vi "User Drivetrain Control.vi"(8 "reinitialize":bool) -> ()   [LabVIEW 2011]
uses:
  <vilib>/Rock Robotics/WPI/RobotDrive/WPI_RobotDriveArcadeDrive_Standard(NoSaturation).vi
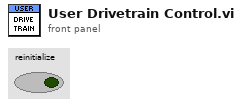
[diagram p1: front panel]
types:
  T1 = typedef "WPI_JoystickDevRef.ctl" = cluster{"Device":T2}
  T2 = typedef "WPI_JoystickDeviceEnum.ctl" = enum16{"USB 1", "USB 2", "USB 3", "USB 4", "Kinect 1", "Kinect 2"}
  T3 = typedef "WPI_JoystickButtonState.ctl" = cluster{"Button 1":bool, "Button 2":bool, "Button 3":bool, "Button 4":bool, "Button 5":bool, "Button 6":bool, "Button 7":bool, "Button 8":bool, "Button 9":bool, "Button 10":bool, "Button 11":bool, "Button 12":bool}
  T4 = cluster{"axis 1 (x)":dbl, "axis 2 (y)":dbl, "axis 3 (throttle)":dbl, "axis 4":dbl, "axis 5":dbl, "axis 6":dbl}
  T5 = typedef "WPI_RobotDriveDevRef.ctl" = cluster{"DevStatus":errorcluster, "Motors[]":T6[], "Square Inputs":bool, "Max Output":dbl, "Isochronous":bool}
  T6 = typedef "WPI_MotorControlDeviceRef.ctl" = cluster{"DeviceStatus":errorcluster, "Type":enum16{"PWM", "CAN"}, "PWM":cluster{"Digital Module":T7, "PWM Channel":T8, "DeadBand":T9}, "CAN":cluster{"Device Number":u8, "Control Mode":T10, "Semaphore":T11, "Max Vout":dbl}, "Invert":bool, "TransformRef":T12, "InvTransformRef":T12}
  T7 = typedef "FPGA_TypedefDigitalModule.ctl" = enum16{"Digital Module 1", "Digital Module 2"}
  T8 = typedef "FPGA_DIOPWMChannel.ctl" = enum8{"PWM 1", "PWM 2", "PWM 3", "PWM 4", "PWM 5", "PWM 6", "PWM 7", "PWM 8", "PWM 9", "PWM 10", "Invalid"}
  T9 = typedef "WPI_PWMDeadband.ctl" = cluster{"Name":string, "maxPositivePwm":i32, "minPositivePwm":i32, "centerPwm":i32, "maxNegativePwm":i32, "minNegativePwm":i32, "angularRange":u16}
  T10 = typedef "WPI_CANJaguar_ControlMode.ctl" = enum8{"Percent VBus", "Current", "Speed", "Position", "Voltage"}
  T11 = typedef "Semaphore RefNum" = refnum<k1>
  T12 = typedef "WPI_PWMTransform_ConPane.ctl" = refnum<vi>
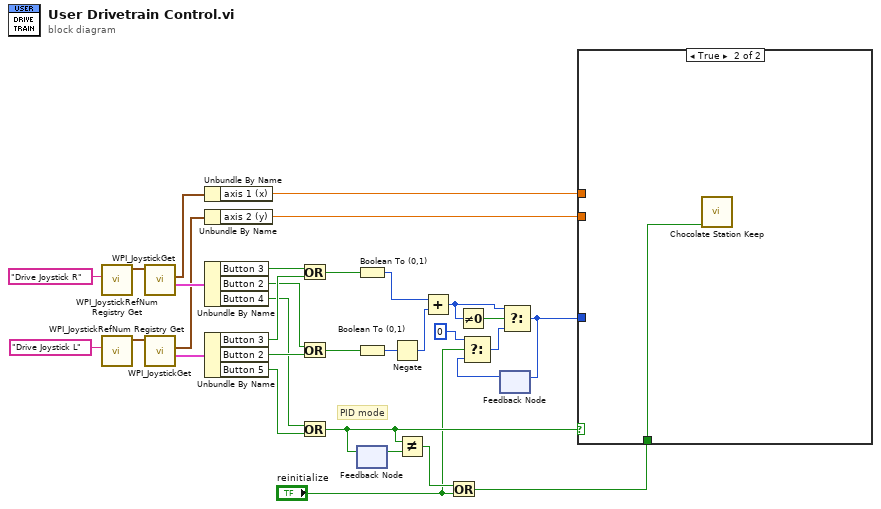
[diagram p0: block diagram]
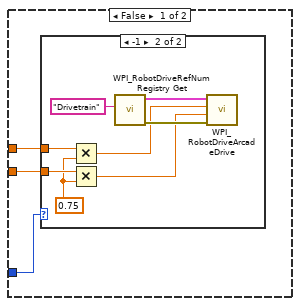
[diagram p2: hidden frame]
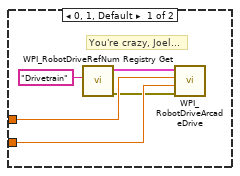
[diagram p3: hidden frame]
diagram:
  # "PID mode"
  n1 = call <vilib>:"WPI_JoystickRefNum Registry Get.vi"("refnum name"="Drive Joystick R") -> ("JoystickDevRef"=w30:T1)  [unwired: 9 in, 1 out]
  n2 = call <vilib>:"WPI_JoystickRefNum Registry Get.vi"("refnum name"="Drive Joystick L") -> ("JoystickDevRef"=w31:T1)  [unwired: 9 in, 1 out]
  n3 = call <vilib>:"WPI_JoystickGet.vi"("JoystickDevRef"=w30) -> ("Buttons"=w28:T3, "Axes"=w22:T4)  [unwired: 4 in, 1 out]
  n4 = call <vilib>:"WPI_JoystickGet.vi"("JoystickDevRef"=w31) -> ("Buttons"=w27:T3, "Axes"=w21:T4)  [unwired: 4 in, 1 out]
  n5 = Unbundle By Name(w22) -> ("axis 1 (x)"=w10:dbl)
  n6 = Unbundle By Name(w21) -> ("axis 2 (y)"=w9:dbl)
  n7 = Unbundle By Name(w28) -> ("Button 3"=w26:bool, "Button 2"=w24:bool, "Button 4"=w20:bool)
  n8 = Unbundle By Name(w27) -> ("Button 3"=w25:bool, "Button 2"=w23:bool, "Button 5"=w19:bool)
  n9 = Or(x=w26, y=w25) -> (x .or. y?=w8:bool)
  n10 = Or(x=w24, y=w23) -> (x .or. y?=w7:bool)
  n11 = Or(x=w20, y=w19) -> (x .or. y?=w16:bool)
  n12 = Boolean To (0,1)(Boolean=w8) -> (0, 1=w12:i16)
  n13 = Boolean To (0,1)(Boolean=w7) -> (0, 1=w14:i16)
  n14 = feedback-in #1(w16) -> ()
  n15 = feedback #1() -> (w17:bool)  [unwired: 1 in]
  n16 = Negate(x=w14) -> (-x=w13:i16)
  n17 = Not Equal?(x=w16, y=w17) -> (x != y?=w15:bool)
  n18 = Add(x=w12, y=w13) -> (x+y=w11:i16)
  n19 = Or(x=w15, y="reinitialize") -> (x .or. y?=w18:bool)
  n20 = Not Equal To 0?(x=w11) -> (x != 0?=w5:bool)
  n21 = feedback #2() -> (w2:i16)  [unwired: 1 in]
  n22 = Select(t=i16 0, s="reinitialize", f=w2) -> (s? t:f=w4:i16)
  n23 = Select(t=w11, s=w5, f=w4) -> (s? t:f=w6:i16)
  n24 = feedback-in #2(w6) -> ()
  n25 = case shown="True" w16 {
    tunnel: w9 -> [w35 _]
    tunnel: w10 -> [w34 _]
    tunnel: w18 -> [_ w49]
    tunnel: w6 -> [w33 _]
    frame False {
      n26 = case shown="-1" w33 {
        tunnel: w35 -> [w40 w43]
        tunnel: w34 -> [w39 w45]
        frame 0, 1, Default {
          # "You're crazy, Joel..."
          n27 = call <vilib>:"WPI_RobotDriveRefNum Registry Get.vi"("refnum name"="Drivetrain") -> ("error out"=w38:errorcluster, "RobotDriveDevRef"=w37:T5)  [unwired: 9 in]
          n28 = call-poly <vilib>:"WPI_RobotDriveArcadeDrive.vi"("error in (no error)"=w38, "Y axis value"=w40, "X axis value"=w39, "RobotDriveDevRef"=w37) -> ()  [unwired: 6 in, 2 out]
        }
        frame -1 {
          w41 = 0.75 ("y")
          n29 = Multiply(x=w45, y=w41) -> (x*y=w44:dbl)
          n30 = Multiply(x=w43, y=w41) -> (x*y=w42:dbl)
          n31 = call <vilib>:"WPI_RobotDriveRefNum Registry Get.vi"("refnum name"="Drivetrain") -> ("error out"=w48:errorcluster, "RobotDriveDevRef"=w47:T5)  [unwired: 9 in]
          n32 = call-poly <vilib>:"WPI_RobotDriveArcadeDrive.vi"("error in (no error)"=w48, "Y axis value"=w42, "X axis value"=w44, "RobotDriveDevRef"=w47) -> ()  [unwired: 6 in, 2 out]
        }
      }
    }
    frame True {
      n33 = call "Chocolate Station Keep.vi"("reinitialize"=w49) -> ()  [unwired: 7 in, 4 out]
    }
  }
